vi "READ_For_Something.vi"(11 "名称":string="data.txt") -> (2 "数组":string[](array[string]), 3 "数组 2":T2(array[cluster]))   [LabVIEW 2014]
doc: "读取txt中存放的测量的数据"
uses:
  <vilib>/Analysis/Matrix/Datatypes/RealMatrix.ctl
  <vilib>/Utility/file.llb/Read From Spreadsheet File (string).vi
  <vilib>/Analysis/Matrix/Numeric/Conversions/Array To Matrix - RA2.vi
  <vilib>/Analysis/Matrix/NI_Matrix.lvlib
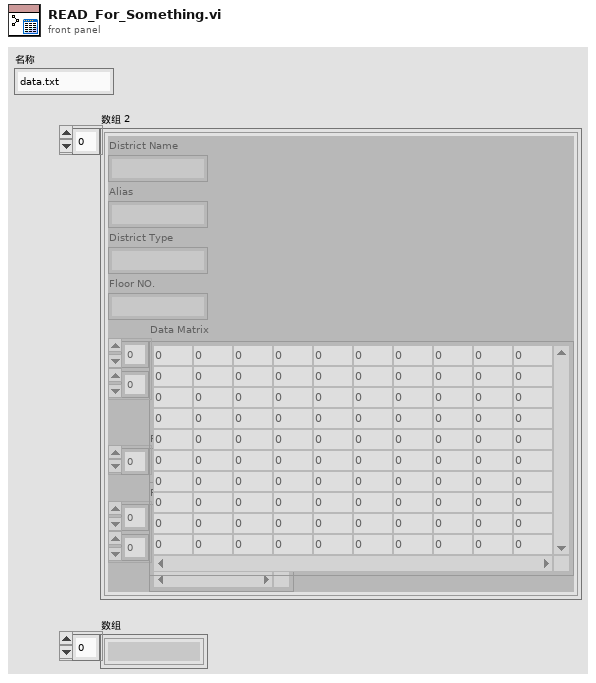
[diagram p1: front panel]
types:
  T1 = typedef "NI_Matrix.lvlib/RealMatrix.ctl" = dbl[][]
  T2 = cluster{"District Name":string, "Alias":string, "District Type":string, "Floor NO.":string, "Data Matrix":T1, "Path array":string[], "Path Coodinate":T1}[]
  T3 = cluster{"District Name":string, "Alias":string, "District Type":string, "Floor NO.":string, "Data Matrix":T1, "Path array":string[], "Path Coodinate":T1}
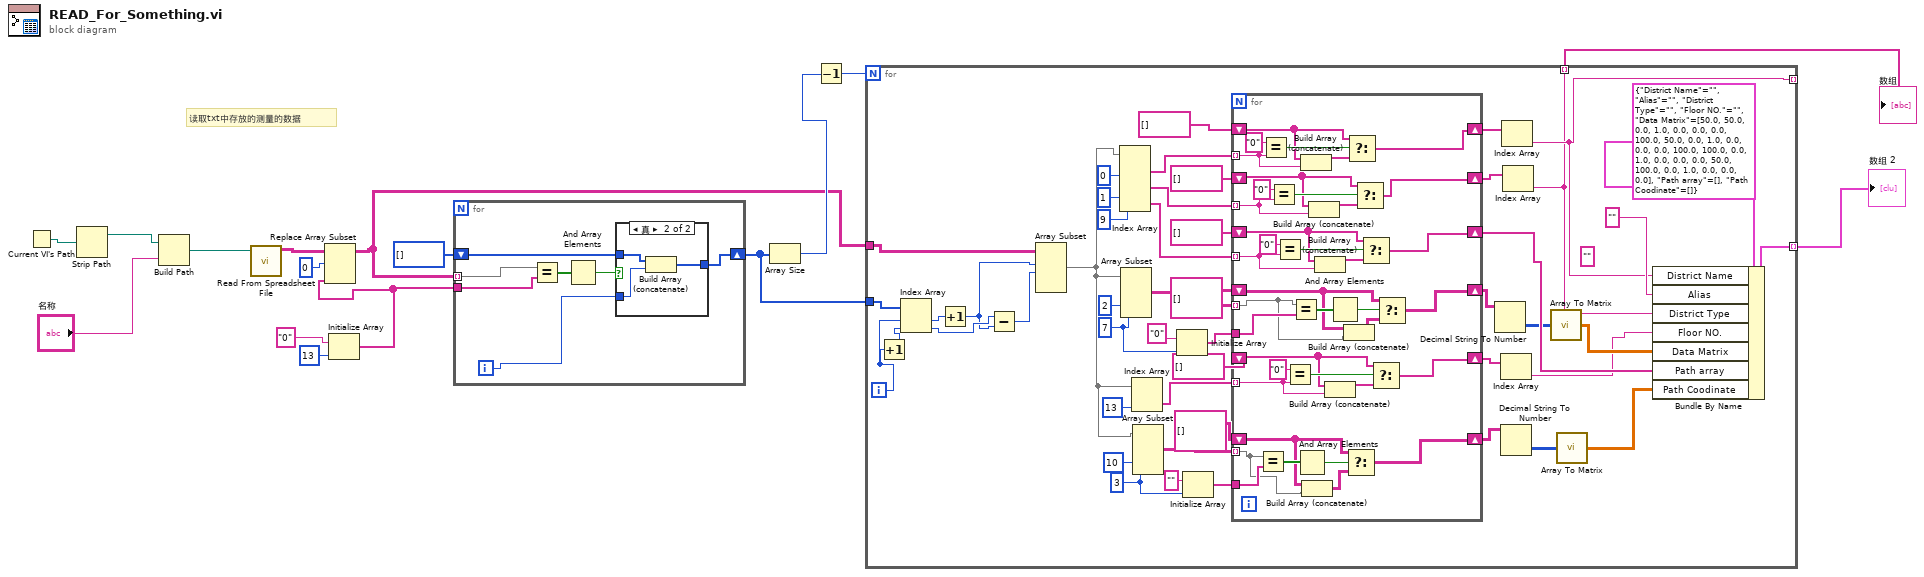
[diagram p0: block diagram]
diagram:
  # "读取txt中存放的测量的数据"
  n1 = Current VI's Path() -> (path=w1:path)
  n2 = Strip Path(path=w1) -> (stripped path=w2:path)  [unwired: 1 out]
  n3 = Build Path(base path=w2, name or relative path="名称") -> (appended path=w4:path)
  n4 = call-poly <vilib>:"Read From Spreadsheet File.vi"("file path (dialog if empty)"=w4) -> ("all rows"=w10:string[][])  [unwired: 6 in, 4 out]
  n5 = Initialize Array("0" ("名称或相对路径"), 13 ("维数大小")) -> (w9:string[])
  n6 = Replace Array Subset(array=w10, new element=w9, index (row)=0 ("索引 (行)")) -> (w12:string[][])  [unwired: 1 in]
  n7 = for {
    tunnel: w12 -> [w23] mode=indexing
    shift-right: [w19] -> w11
    shift-left: i32[] [] -> [w18]
    tunnel: w9 -> [w17]
    i -> [w20]
    n8 = Equal?(x=w23, y=w17) -> (x = y?=w22:bool[])
    n9 = And Array Elements(Boolean array=w22) -> (logical AND=w21:bool)
    n10 = case shown="真" w21 {
      tunnel: w20 -> [_ w27]
      tunnel: [w24 w26] -> w19
      tunnel: w18 -> [w24 w25]
      frame False {
      }
      frame True {
        n11 = Build Array (concatenate)(w25, w27) -> (w26:i32[])
      }
    }
  }
  n12 = Array Size(array=w11) -> (size(s)=w14:i32)
  n13 = Decrement(x=w14) -> (x-1=w13:i32)
  n14 = for {
    N: w13 -> [_]
    tunnel: w12 -> [w72]
    tunnel: w11 -> [w76]
    tunnel: [w47] -> w15 mode=indexing
    tunnel: [w39] -> _ mode=indexing
    tunnel: [w28] -> w16 mode=indexing
    i -> [w74]
    w35 = 3 ("长度")
    (unwired) "" ("Floor NO.")
    w57 = 7 ("长度")
    n15 = Increment(x=w74) -> (x+1=w75:i32)
    n16 = Index Array(array=w76, index #1=w74, index #2=w75) -> (element #1=w73:i32, element #2=w71:i32)
    n17 = Increment(x=w73) -> (x+1=w70:i32)
    n18 = Subtract(x=w71, y=w70) -> (x-y=w69:i32)
    n19 = Array Subset(array=w72, index (row)=w70, length (row)=w69) -> (w38:string[][])  [unwired: 2 in]
    n20 = Index Array(array=w38, index (col) #1=0 ("禁用的索引 (列)"), index (col) #2=1 ("索引 (列)"), index (col) #3=9 ("索引 (列)")) -> (element #1=w64:string[], element #2=w63:string[], element #3=w62:string[])  [unwired: 3 in]
    n21 = Array Subset(array=w38, index (col)=2 ("索引"), length (col)=w57) -> (w45:string[][])  [unwired: 2 in]
    n22 = Index Array(array=w38, index (col)=13 ("禁用的索引 (列)")) -> (element=w43:string[])  [unwired: 1 in]
    n23 = Array Subset(array=w38, index (col)=10 ("索引"), length (col)=w35) -> (w36:string[][])  [unwired: 2 in]
    n24 = Initialize Array("0" ("名称或相对路径"), w57) -> (w56:string[])
    n25 = Initialize Array("" ("元素"), w35) -> (w33:string[])
    n26 = for {
      tunnel: w64 -> [w112] mode=indexing
      tunnel: w63 -> [w105] mode=indexing
      tunnel: w62 -> [w99] mode=indexing
      shift-right: [w110] -> w52
      shift-left: string[] [] -> [w109]
      shift-right: [w104] -> w51
      shift-left: string[] [] -> [w103]
      shift-right: [w98] -> w50
      shift-left: string[] [] -> [w97]
      tunnel: w45 -> [w90] mode=indexing
      tunnel: w56 -> [w93]
      shift-right: [w96] -> w54
      shift-left: string[][] [] -> [w91]
      tunnel: w43 -> [w86] mode=indexing
      shift-right: [w85] -> w41
      shift-left: string[] [] -> [w84]
      tunnel: w36 -> [w79] mode=indexing
      tunnel: w33 -> [w83]
      shift-right: [w80] -> w30
      shift-left: string[][] [] -> [w77]
      n27 = Equal?(x=w79, y=w83) -> (x = y?=w82:bool[])
      n28 = Equal?(x="0", y=w112) -> (x = y?=w113:bool)
      n29 = Equal?(x="0", y=w105) -> (x = y?=w107:bool)
      n30 = Equal?(x="0", y=w99) -> (x = y?=w101:bool)
      n31 = Equal?(x="0", y=w86) -> (x = y?=w88:bool)
      n32 = Equal?(x=w90, y=w93) -> (x = y?=w95:bool[])
      n33 = And Array Elements(Boolean array=w82) -> (logical AND=w81:bool)
      n34 = Build Array (concatenate)(w109, w112) -> (w111:string[])
      n35 = Build Array (concatenate)(w77, w79) -> (w78:string[][])
      n36 = Build Array (concatenate)(w103, w105) -> (w108:string[])
      n37 = Build Array (concatenate)(w97, w99) -> (w100:string[])
      n38 = Build Array (concatenate)(w84, w86) -> (w89:string[])
      n39 = And Array Elements(Boolean array=w95) -> (logical AND=w94:bool)
      n40 = Build Array (concatenate)(w91, w90) -> (w92:string[][])
      n41 = Select(t=w77, s=w81, f=w78) -> (s? t:f=w80:string[][])
      n42 = Select(t=w109, s=w113, f=w111) -> (s? t:f=w110:string[])
      n43 = Select(t=w103, s=w107, f=w108) -> (s? t:f=w104:string[])
      n44 = Select(t=w97, s=w101, f=w100) -> (s? t:f=w98:string[])
      n45 = Select(t=w84, s=w88, f=w89) -> (s? t:f=w85:string[])
      n46 = Select(t=w91, s=w94, f=w92) -> (s? t:f=w96:string[][])
    }
    n47 = Decimal String To Number(string=w54) -> (number=w49:i32[][])  [unwired: 2 in, 1 out]
    n48 = Index Array(array=w41) -> (element=w40:string)  [unwired: 1 in]
    n49 = Decimal String To Number(string=w30) -> (number=w31:i32[][])  [unwired: 2 in, 1 out]
    n50 = Index Array(array=w52) -> (element=w39:string)  [unwired: 1 in]
    n51 = Index Array(array=w51) -> (element=w28:string)  [unwired: 1 in]
    n52 = call-poly <vilib>:"Array To Matrix.vi"("Real 2D Array"=w49) -> ("Real Matrix"=w48:T1)
    n53 = call-poly <vilib>:"Array To Matrix.vi"("Real 2D Array"=w31) -> ("Real Matrix"=w29:T1)
    n54 = Bundle By Name(cluster=T3 {"District Name"="", "Alias"="", "District Type"="", "Floor NO."="", "Data Matrix"=[[50.0, 50.0, 0.0, 1.0, 0.0, 0.0, 0.0], [100.0, 50.0, 0.0, 1.0, 0.0, 0.0, 0.0], [100.0, 100.0, 0.0, 1.0, 0.0, 0.0, 0.0], [50.0, 100.0, 0.0, 1.0, 0.0, 0.0, 0.0]], "Path array"=[], "Path Coodinate"=[]} ("输入簇"), "District Name"=w39, "Alias"="", "District Type"=w28, "Floor NO."=w40, "Data Matrix"=w48, "Path array"=w50, "Path Coodinate"=w29) -> (w47:T3)
  }
  "数组" <- w16
  "数组 2" <- w15
